vi "Pause VI.vi"(8 "error in (no error)":errorcluster, 11 "VI in":refnum<vi>) -> (0 "error out":errorcluster, 3 "VI out":refnum<vi>)   [LabVIEW 2011]
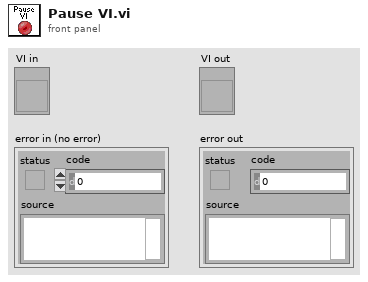
[diagram p1: front panel]
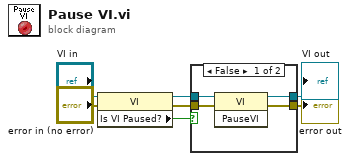
[diagram p0: block diagram]
diagram:
  n1 = property class="VI"(reference="VI in", error in="error in (no error)") -> (reference out=w4:refnum<vi>, error out=w6:errorcluster, "Is VI Paused?"=w7:bool)
  n2 = case shown="False" w7 {
    tunnel: [w11 w12] -> w2
    tunnel: [w10 w13] -> w3
    tunnel: w4 -> [w9 w13]
    tunnel: w6 -> [w8 w12]
    frame False {
      n3 = invoke class="VI" method="PauseVI"(reference=w9, error in=w8) -> (reference out=w10:refnum<vi>, error out=w11:errorcluster)  [unwired: 1 in, 1 out]
    }
    frame True {
    }
  }
  "VI out" <- w3
  "error out" <- w2
